vi "V7310.Job.Main.Variables.Get.vi"(6 "timeout ms (5000)":i32=5000, 8 "error in":errorcluster, 11 "Connection in":refnum<k5>) -> (0 "error out":errorcluster, 2 "VarNames":T1[](array[typedef]), 3 "Connection out":refnum<k5>)   [LabVIEW 2016]
uses:
  LowLevel/V7310.Job.Variable.ctl
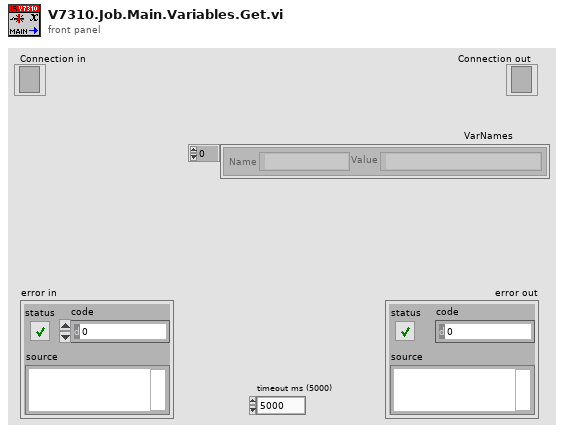
[diagram p1: front panel]
types:
  T1 = typedef "V7310.Job.Variable.ctl" = cluster{"Name":string, "Value":string}
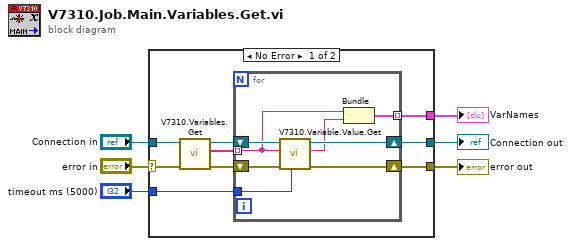
[diagram p0: block diagram]
diagram:
  n1 = case shown="No Error" "error in" {
    selector: "error in" -> [w11 w23]
    tunnel: "Connection in" -> [w12 w24]
    tunnel: [w14 w24] -> w5
    tunnel: "timeout ms (5000)" -> [w10 _]
    tunnel: [w9 w23] -> w2
    tunnel: [w7 _] -> w1
    frame No Error {
      n2 = call "V7310.Variables.Get.vi"("error in"=w11, "Connection in"=w12) -> ("error out"=w13:errorcluster, "Variables"=w8:string[], "Connection out"=w14:refnum<k5>)  [unwired: 7 in]
      n3 = for {
        tunnel: w10 -> [w20]
        shift-right: [w19] -> w9
        shift-left: w13 -> [w22]
        shift-right: [w18] -> _
        shift-left: w14 -> [w21]
        tunnel: w8 -> [w17] mode=indexing
        tunnel: [w15] -> w7 mode=indexing
        n4 = call "V7310.Variable.Value.Get.vi"("timeout ms (5000)"=w20, "error in"=w22, "Variable"=w17, "Connection in"=w21) -> ("error out"=w19:errorcluster, "Value"=w16:string, "Connection out"=w18:refnum<k5>)  [unwired: 5 in]
        n5 = Bundle(w17, "Value"=w16) -> (w15:cluster{string, "Value":string})  [unwired: 1 in]
      }
    }
    frame Error {
    }
  }
  "Connection out" <- w5
  "error out" <- w2
  "VarNames" <- w1
